vi "Sergey_Koshelev_Ex 2-2 C to F.vi"(0 "Deg C":dbl) -> (1 "Deg F":dbl)   [LabVIEW 2024]
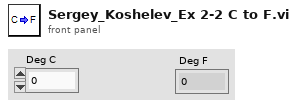
[diagram p1: front panel]
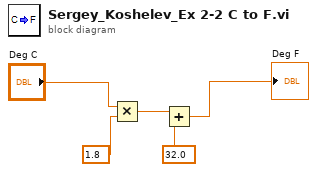
[diagram p0: block diagram]
diagram:
  n1 = Multiply(x="Deg C", y=1.8) -> (x*y=w3:dbl)
  n2 = Add(x=w3, y=32.0) -> (x+y=→"Deg F":dbl)
